vi "Boolean_NoError.vi"() -> ()   [LabVIEW 2017, in "Assertion.Tests.lvlib" / "AssertIsBoolean.lvlib"]
uses:
  AssertIsBoolean.lvlib
  Assertion/Assertion.lvlib
panel:
  out "error out":errorcluster
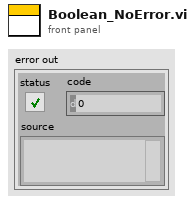
[diagram p1: front panel]
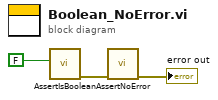
[diagram p0: block diagram]
diagram:
  n1 = call "AssertIsBoolean.vi"("Actual"=FALSE) -> ("error out"=w2:errorcluster)  [unwired: 10 in]
  n2 = call "AssertNoError.vi"("error in (no error)"=w2) -> ("error out"=→"error out":errorcluster)  [unwired: 10 in]
